vi "Frame Operation.vi"() -> ()   [LabVIEW 2017, in "Expansion.lvclass"]
uses:
  Expansion.lvclass
  Type Defs/Expansion Queue Element.ctl
  Type Defs/Expansion State.ctl
panel:
  in  "Stop":bool
  in  "Start":bool
  out "Expansion Recipe":string
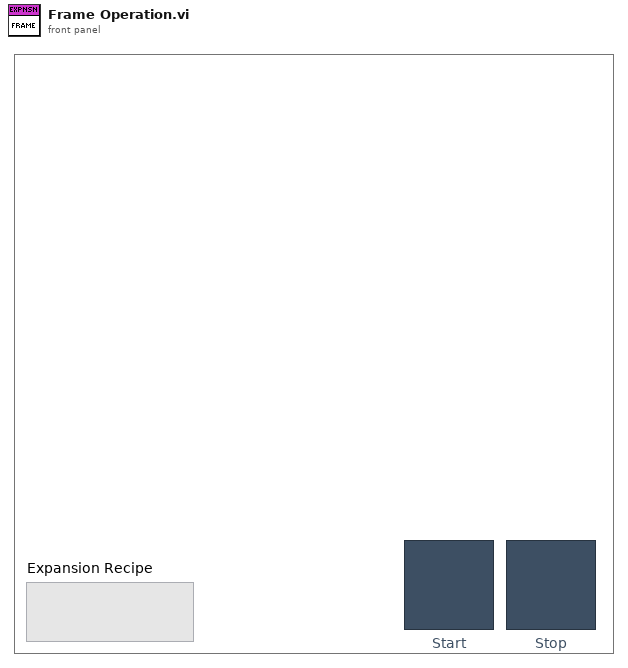
[diagram p1: front panel]
types:
  T1 = typedef "Expansion.lvclass/Expansion Queue Element.ctl" = cluster{"State":T2, "Variant":variant}
  T2 = typedef "Expansion.lvclass/Expansion State.ctl" = enum16{"Init", "Go", "Stop", "Idle", "Error", "Shutdown"}
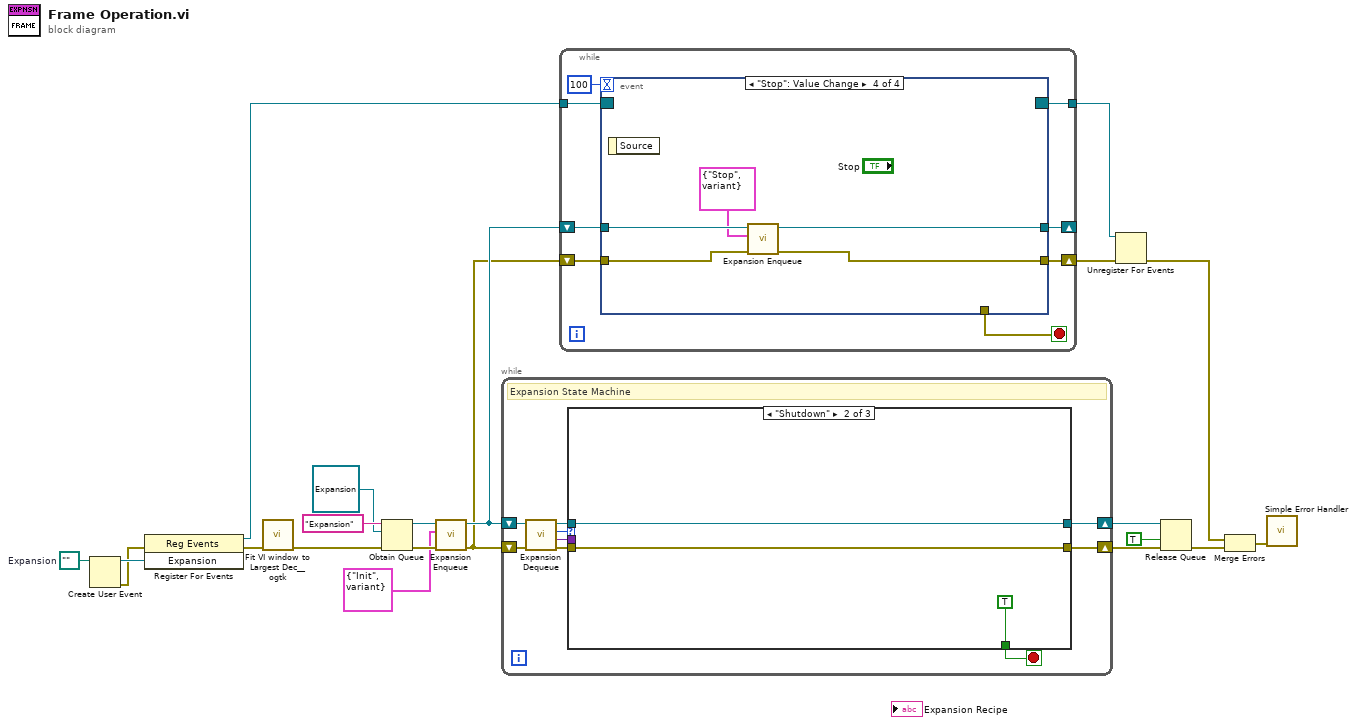
[diagram p0: block diagram]
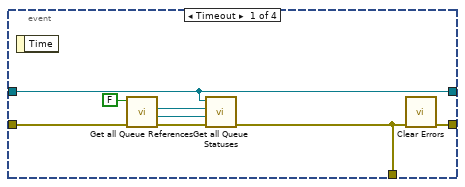
[diagram p2: hidden frame]
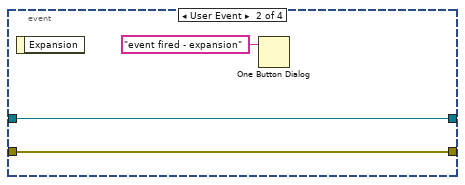
[diagram p3: hidden frame]
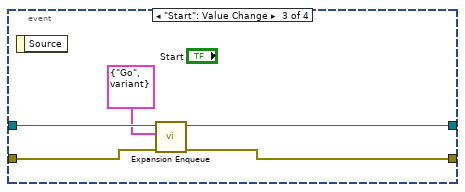
[diagram p4: hidden frame]
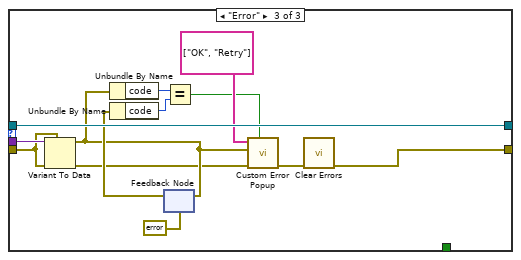
[diagram p6: hidden frame]
diagram:
  w9 = path ""  # Expansion
  n1 = Create User Event(user event datatype=w9) -> (user event=w8:refnum<user-event>, error out=w6:errorcluster)  [unwired: 1 in]
  n2 = register-events(error in=w6, w8) -> (reference out=w7:refnum<event-registration>, error out=w5:errorcluster)  [unwired: 1 in]
  n3 = call "Fit VI window to Largest Dec__ogtk.vi"("error in (no error)"=w5) -> ("error out"=w16:errorcluster)  [unwired: 5 in, 1 out]
  n4 = Obtain Queue(name (unnamed)="Expansion", element data type=refnum<class "Expansion.lvclass"> refnum ("Expansion.lvclass"), error in (no error)=w16) -> (queue out=w18:refnum<queue>, error out=w17:errorcluster)  [unwired: 2 in, 1 out]
  n5 = call "Expansion Enqueue.vi"("error in (no error)"=w17, "Expansion Queue Element"=T1 {"State"=enum."Init", "Variant"=variant}, "Queue in"=w18) -> ("error out"=w11:errorcluster, "Queue out"=w12:refnum<queue>)  [unwired: 7 in]
  n6 = while {
    shift-right: [w26] -> w20
    shift-left: w11 -> [w29]
    shift-right: [w24] -> w21
    shift-left: w12 -> [w30]
    stop <- w25 stop-if-true
    # "Expansion State Machine"
    n7 = call "Expansion Dequeue.vi"("error in (no error)"=w29, "Queue in"=w30) -> ("error out"=w27:errorcluster, "Data"=w22:variant, "State"=w23:T2, "Queue out"=w28:refnum<queue>)  [unwired: 6 in]
    n8 = case shown="\"Shutdown\"" w23 {
      tunnel: w28 -> [w31 w34 w48]
      tunnel: w27 -> [w32 w35 w38]
      tunnel: [w32 w35 w45] -> w26
      tunnel: [_ TRUE _] -> w25
      tunnel: [w31 w34 w48] -> w24
      tunnel: w22 -> [_ _ w39]
      frame "Idle", Default {
      }
      frame "Shutdown" {
      }
      frame "Error" {
        n9 = Variant To Data(error in=w38, type=w38, Variant=w39) -> (data=w37:errorcluster, error out=w36:errorcluster)
        n10 = Unbundle By Name(w37) -> ("code"=w43:i32)
        n11 = feedback-in #1(w37) -> ()
        n12 = feedback #1(errorcluster {"status"=FALSE, "code"=0, "source"=""} ("error out")) -> (w44:errorcluster)
        n13 = Unbundle By Name(w44) -> ("code"=w42:i32)
        n14 = Equal?(x=w43, y=w42) -> (x = y?=w41:bool)
        n15 = call "Custom Error Popup.vi"("Repeated error?"=w41, "VI Error in"=w36, "Error to display"=w37, "Button Labels"=string[] ["OK", "Retry"]) -> ("error out"=w47:errorcluster)  [unwired: 6 in, 1 out]
        n16 = call <vilib>:"Clear Errors.vi"("error in (no error)"=w47) -> ("error out"=w45:errorcluster)  [unwired: 5 in, 1 out]
      }
    }
  }
  n17 = while {
    shift-right: [w53] -> w4
    shift-left: w11 -> [w55]
    shift-right: [w52] -> _
    shift-left: w12 -> [w56]
    tunnel: w7 -> [w50]
    tunnel: [w49] -> w3
    stop <- w54 stop-if-true
    n18 = event shown="[3] \"Stop\": Value Change" {
      selector: w50 -> [_ _ _ _]
      dyn-events: [_ _ _ _] -> w49
      timeout: 100 -> [_ _ _ _]
      tunnel: w56 -> [w58 w66 w72 w77]
      tunnel: w55 -> [w60 w67 w70 w75]
      tunnel: [w61 _ _ _] -> w54
      tunnel: [w57 w67 w69 w74] -> w53
      tunnel: [w58 w66 w71 w76] -> w52
      event Timeout {
        n19 = event-data() -> ()  [unwired: 1 in, 1 out]
        n20 = call "Get all Queue References.vi"("error in (no error)"=w60, "create if not found? (F)"=FALSE ("create if not found? (T)")) -> ("error out"=w62:errorcluster, "Recipes Queue"=w63:refnum<queue>, "Saturation Queue"=w64:refnum<queue>)  [unwired: 6 in, 1 out]
        n21 = call "Get all Queue Statuses.vi"("error in (no error)"=w62, "Recipes Queue"=w63, "Saturation Queue"=w64, "Queue in"=w58) -> ("error out"=w61:errorcluster)  [unwired: 7 in]
        n22 = call <vilib>:"Clear Errors.vi"("error in (no error)"=w61) -> ("error out"=w57:errorcluster)  [unwired: 5 in, 1 out]
      }
      event User Event {
        n23 = event-data() -> ()  [unwired: 1 in, 1 out]
        n24 = One Button Dialog(message="event fired - expansion") -> ()  [unwired: 1 in, 1 out]
      }
      event "Start": Value Change {
        n25 = event-data() -> ()  [unwired: 1 in, 1 out]
        n26 = call "Expansion Enqueue.vi"("error in (no error)"=w70, "Expansion Queue Element"=T1 {"State"=enum."Go", "Variant"=variant}, "Queue in"=w72) -> ("error out"=w69:errorcluster, "Queue out"=w71:refnum<queue>)  [unwired: 7 in]
      }
      event "Stop": Value Change {
        n27 = event-data() -> ()  [unwired: 1 in, 1 out]
        n28 = call "Expansion Enqueue.vi"("error in (no error)"=w75, "Expansion Queue Element"=T1 {"State"=enum."Stop", "Variant"=variant}, "Queue in"=w77) -> ("error out"=w74:errorcluster, "Queue out"=w76:refnum<queue>)  [unwired: 7 in]
      }
    }
  }
  n29 = Unregister For Events(event registration refnum=w3, error in=w4) -> (error out=w1:errorcluster)
  n30 = Release Queue(queue=w21, force destroy? (F)=TRUE, error in (no error)=w20) -> (error out=w13:errorcluster)  [unwired: 2 out]
  n31 = Merge Errors(w1, w13) -> (w2:errorcluster)
  n32 = call <vilib>:"Simple Error Handler.vi"("error in (no error)"=w2) -> ()  [unwired: 4 in, 5 out]
